vi "Read Menu Reference.vi"(8 "error in (no error)":errorcluster, 11 "MenuButton in":refnum<class "MenuButton.lvclass">) -> (0 "error out":errorcluster, 2 "Menu Reference":refnum<vi>, 3 "MenuButton out":refnum<class "MenuButton.lvclass">)   [LabVIEW 2017, in "MenuButtons.lvlib" / "MenuButton.lvclass"]
uses:
  MenuButton.lvclass
  MenuButton.lvclass/MenuButton.ctl
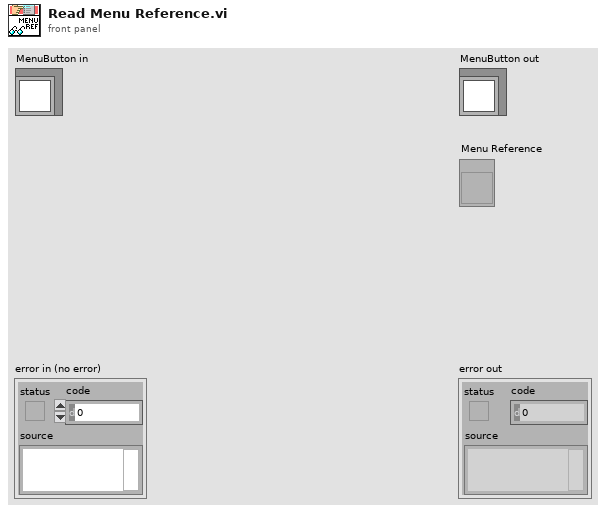
[diagram p1: front panel]
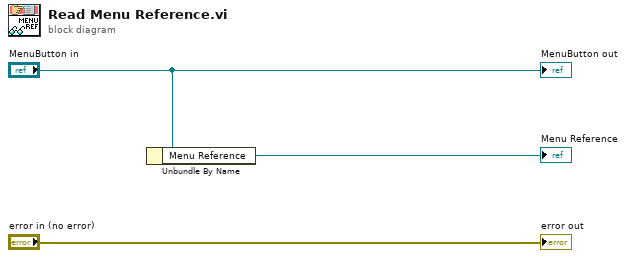
[diagram p0: block diagram]
diagram:
  n1 = Unbundle By Name("MenuButton in") -> ("Menu Reference"=→"Menu Reference":refnum<vi>)
  "error out" <- "error in (no error)"
  "MenuButton out" <- "MenuButton in"
